vi "AlliGator Source Image ROI Storage [PM].vi"   [LabVIEW 2021, in "AlliGator ROIs.lvlib"]
doc: "Handles single or multiple Source Image ROI(s) storage."
uses:
  AlliGator ROIs.lvlib
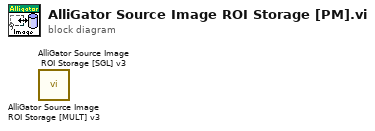
[diagram p0: block diagram]
diagram:
  n1 = call "AlliGator Source Image ROI Storage [MULT] v3.vi"() -> ()  [unwired: 6 in, 6 out]
  n2 = call "AlliGator Source Image ROI Storage [SGL] v3.vi"() -> ()  [unwired: 5 in, 7 out]
